vi "thermalCamera.vi"() -> ()   [LabVIEW 2025]
panel:
  out "Image":T1(plugin-control)
  out "IP address":string
  in  "Stop Button":bool
  out "Output":string
  in  "Flag":bool
  in  "Stop recording":bool
  in  "Stop Preview":bool
  in  "Server Path":path
  in  "Focus":dbl(slide) scale=0.0..100.0
  in  "Record":bool
  in  "Connect Server":bool
  out "?":string
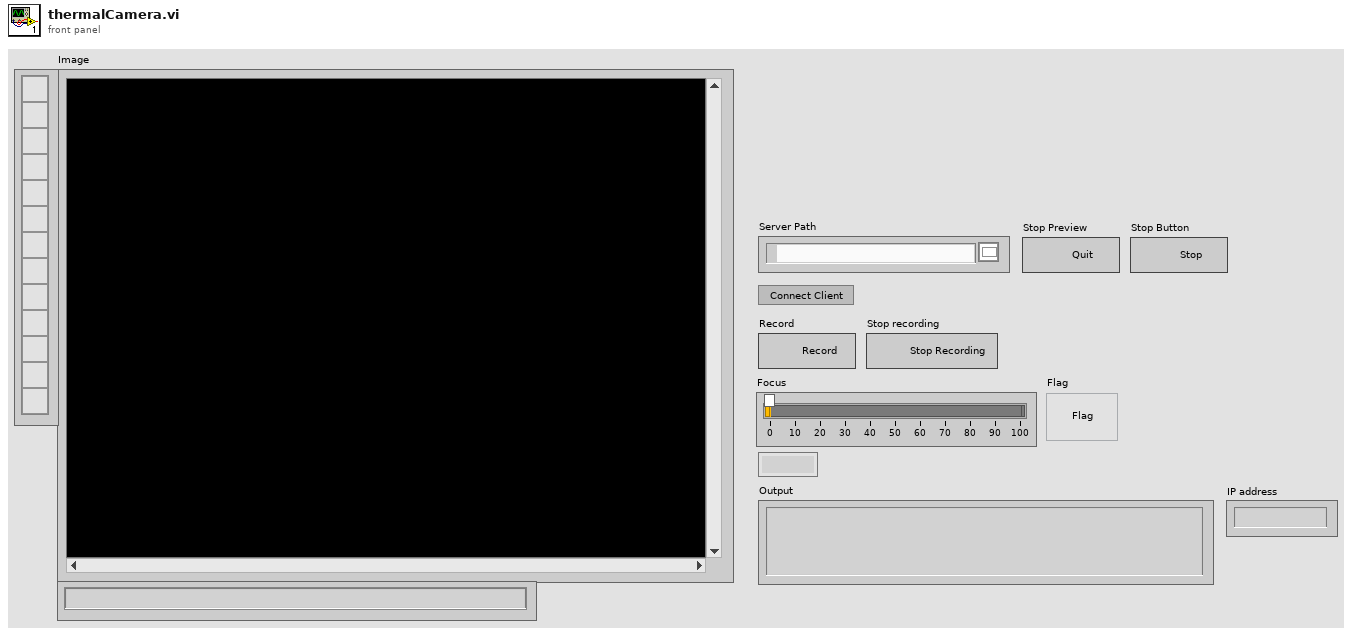
[diagram p1: front panel]
types:
  T1 = typedef "IMAQ Image.ctl" = refnum<image>
  T2 = typedef "Image Type" = u32
  T3 = enum16{"open", "replace", "create", "open or create", "replace or create", "replace or create with confirmation"}
  T4 = enum16{"big-endian, network order", "native, host order", "little-endian"}
  T5 = enum16{"Standard", "Buffered", "CRLF", "Immediate"}
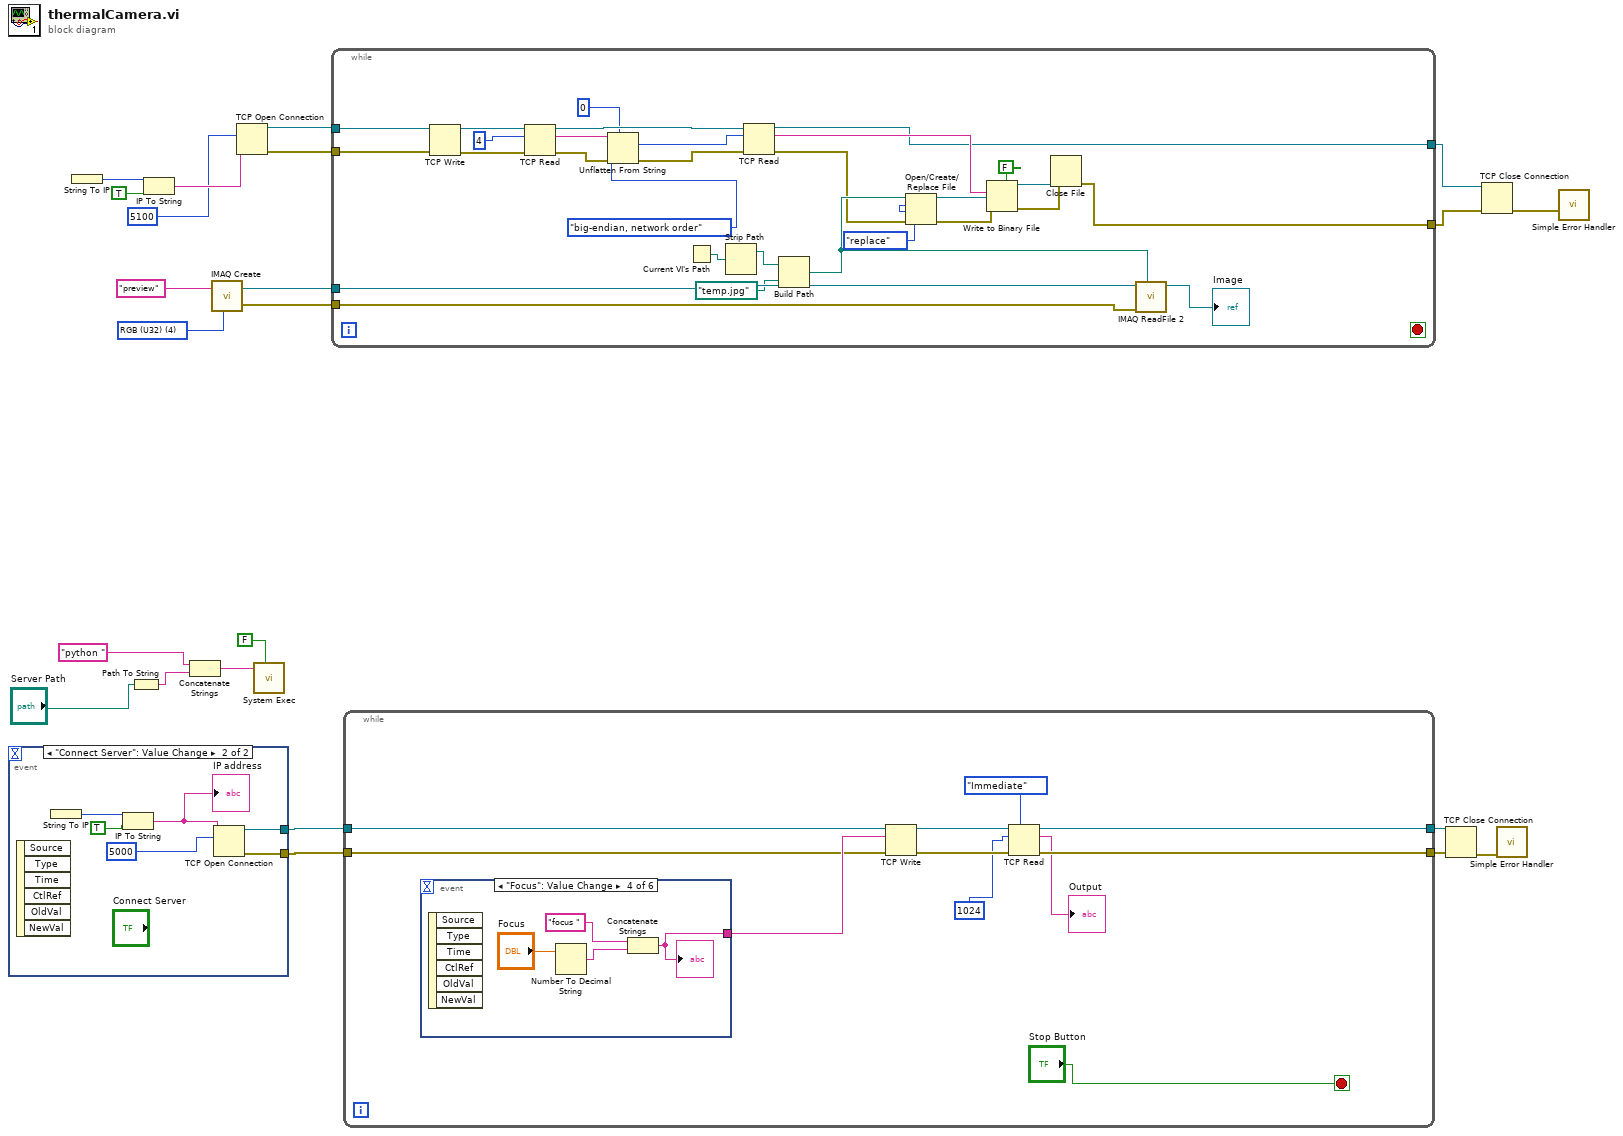
[diagram p0: block diagram]
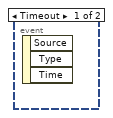
[diagram p2: hidden frame]
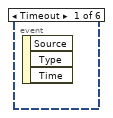
[diagram p3: hidden frame]
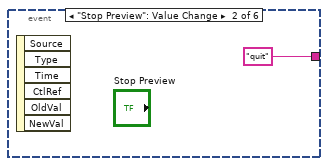
[diagram p4: hidden frame]
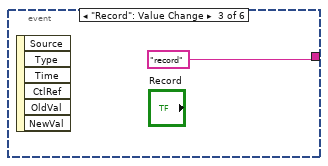
[diagram p5: hidden frame]
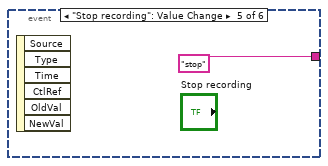
[diagram p6: hidden frame]
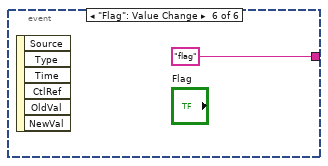
[diagram p7: hidden frame]
diagram:
  w7 = T2 4 items=["Grayscale (U8)", "Grayscale (I16)", "Grayscale (SGL)", "Complex (CSG)", "RGB (U32)", "HSL (U32)", "RGB (U64)", "Grayscale (U16)"] ("Image Type")
  n1 = event shown="[1] \"Connect Server\": Value Change" {
    selector: _ -> [_ _]
    dyn-events: _ -> [_ _]
    timeout: _ -> [_ _]
    tunnel: [_ w28] -> w18
    tunnel: [_ w27] -> w17
    event Timeout {
      n2 = event-data() -> ()  [unwired: 1 in, 3 out]
    }
    event "Connect Server": Value Change {
      n3 = event-data() -> ()  [unwired: 1 in, 6 out]
      n4 = String To IP() -> (0:w26:u32)  [unwired: 1 in]
      n5 = IP To String(1:TRUE ("dot notation? (F)"), 2:w26) -> (0:w24:string)
      "IP address" <- w24
      n6 = TCP Open Connection(address=w24, remote port or service name=u16 5000) -> (connection ID=w27:refnum<k5>, error out=w28:errorcluster)  [unwired: 3 in]
    }
  }
  n7 = String To IP() -> (0:w12:u32)  [unwired: 1 in]
  n8 = Path To String(path="Server Path") -> (string=w19:string)
  n9 = IP To String(1:TRUE ("dot notation? (F)"), 2:w12) -> (0:w13:string)
  n10 = Concatenate Strings("python " ("string"), w19) -> (w15:string)
  n11 = call "IMAQ Create"("Image Name"="preview", "Image Type"=w7) -> ("New Image"=w5:T1, "error out"=w6:errorcluster)  [unwired: 3 in]
  n12 = TCP Open Connection(address=w13, remote port or service name=u16 5100) -> (connection ID=w3:refnum<k5>, error out=w4:errorcluster)  [unwired: 3 in]
  n13 = call <vilib>:"System Exec.vi"("wait until completion? (T)"=FALSE, "command line"=w15) -> ()  [unwired: 6 in, 4 out]
  n14 = while {
    tunnel: w6 -> [w41]
    tunnel: w5 -> [w40]
    tunnel: w4 -> [w33]
    tunnel: w3 -> [w32]
    tunnel: [w31] -> w2
    tunnel: [w30] -> w1
    stop <- _ stop-if-true
    n15 = TCP Write(connection ID=w32, error in (no error)=w33) -> (connection ID out=w42:refnum<k5>, error out=w43:errorcluster)  [unwired: 2 in, 1 out]
    n16 = TCP Read(connection ID=w42, bytes to read=4, error in (no error)=w43) -> (connection ID out=w45:refnum<k5>, data out=w44:string, error out=w47:errorcluster)  [unwired: 2 in]
    n17 = Unflatten From String(type=0, binary string=w44, byte order (0:big-endian, network order)=T4."big-endian, network order", error in (no error)=w47) -> (value=w46:i32, error out=w48:errorcluster)  [unwired: 1 in, 1 out]
    n18 = Current VI's Path() -> (path=w49:path)
    n19 = Strip Path(path=w49) -> (stripped path=w50:path)  [unwired: 1 out]
    n20 = TCP Read(connection ID=w45, bytes to read=w46, error in (no error)=w48) -> (connection ID out=w30:refnum<k5>, data out=w52:string, error out=w54:errorcluster)  [unwired: 2 in]
    n21 = Build Path(base path=w50, name or relative path=path "temp.jpg") -> (appended path=w57:path)
    n22 = Open/Create/Replace File(file path (use dialog)=w57, error in=w54, operation (0:open)=T3."replace") -> (refnum out=w51:refnum<file>, error out=w55:errorcluster)  [unwired: 3 in, 1 out]
    n23 = Write to Binary File(file (use dialog)=w51, data=w52, error in=w55, 5:FALSE ("prepend array or string size? (T)")) -> (refnum out=w53:refnum<file>, error out=w56:errorcluster)  [unwired: 2 in, 1 out]
    n24 = Close File(refnum=w53, error in=w56) -> (error out=w31:errorcluster)  [unwired: 1 out]
    n25 = call "IMAQ ReadFile 2"("File Path"=w57, "error in (no error)"=w41, "Image"=w40) -> ("Image Out"=→"Image":T1)  [unwired: 4 in, 4 out]
  }
  n26 = while {
    tunnel: [w68] -> w23
    tunnel: [w66] -> w22
    tunnel: w18 -> [w64]
    tunnel: w17 -> [w63]
    stop <- "Stop Button" stop-if-true
    n27 = event shown="[3] \"Focus\": Value Change" {
      selector: _ -> [_ _ _ _ _ _]
      dyn-events: _ -> [_ _ _ _ _ _]
      timeout: _ -> [_ _ _ _ _ _]
      tunnel: [_ "quit" "record" w73 "stop" "flag"] -> w65
      event Timeout {
        n28 = event-data() -> ()  [unwired: 1 in, 3 out]
      }
      event "Stop Preview": Value Change {
        n29 = event-data() -> ()  [unwired: 1 in, 6 out]
      }
      event "Record": Value Change {
        n30 = event-data() -> ()  [unwired: 1 in, 6 out]
      }
      event "Focus": Value Change {
        n31 = event-data() -> ()  [unwired: 1 in, 6 out]
        n32 = Number To Decimal String(number="Focus") -> (decimal integer string=w75:string)  [unwired: 1 in]
        n33 = Concatenate Strings("focus ", w75) -> (w73:string)
        "?" <- w73
      }
      event "Stop recording": Value Change {
        n34 = event-data() -> ()  [unwired: 1 in, 6 out]
      }
      event "Flag": Value Change {
        n35 = event-data() -> ()  [unwired: 1 in, 6 out]
      }
    }
    n36 = TCP Write(connection ID=w63, data in=w65, error in (no error)=w64) -> (connection ID out=w67:refnum<k5>, error out=w69:errorcluster)  [unwired: 1 in, 1 out]
    n37 = TCP Read(connection ID=w67, bytes to read=1024, error in (no error)=w69, 7:T5."Immediate" ("mode (standard)")) -> (connection ID out=w66:refnum<k5>, data out=→"Output":string, error out=w68:errorcluster)  [unwired: 1 in]
  }
  n38 = TCP Close Connection(connection ID=w22, error in (no error)=w23) -> (error out=w21:errorcluster)  [unwired: 1 in, 1 out]
  n39 = TCP Close Connection(connection ID=w1, error in (no error)=w2) -> (error out=w9:errorcluster)  [unwired: 1 in, 1 out]
  n40 = call <vilib>:"Simple Error Handler.vi"("error in (no error)"=w21) -> ()  [unwired: 4 in, 5 out]
  n41 = call <vilib>:"Simple Error Handler.vi"("error in (no error)"=w9) -> ()  [unwired: 4 in, 5 out]
